vi "labVIEW_combinatie.vi"() -> ()   [LabVIEW 2019]
panel:
  in  "linksachter":bool
  in  "rechtsachter":bool
  in  "rechtsvooruit":bool
  in  "linksvooruit":bool
  in  "rechts":bool
  in  "links":bool
  out "port":u16
  in  "stop 2":bool
  out "data out":string
  in  "achteruit":bool
  in  "vooruit":bool
  in  "stop":bool
  # "sender"
  # "receiver"
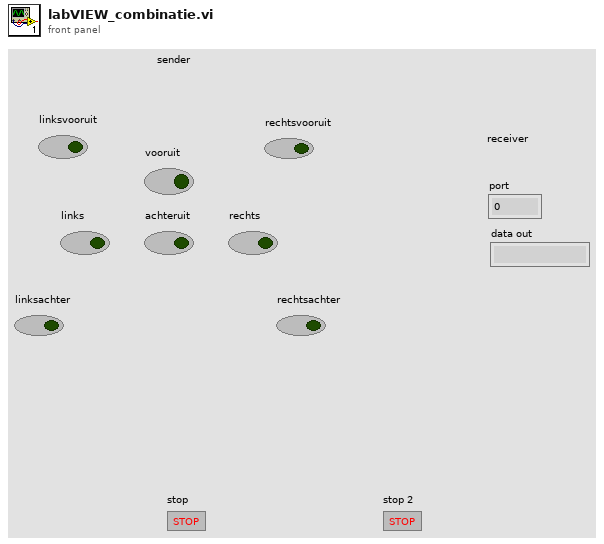
[diagram p1: front panel]
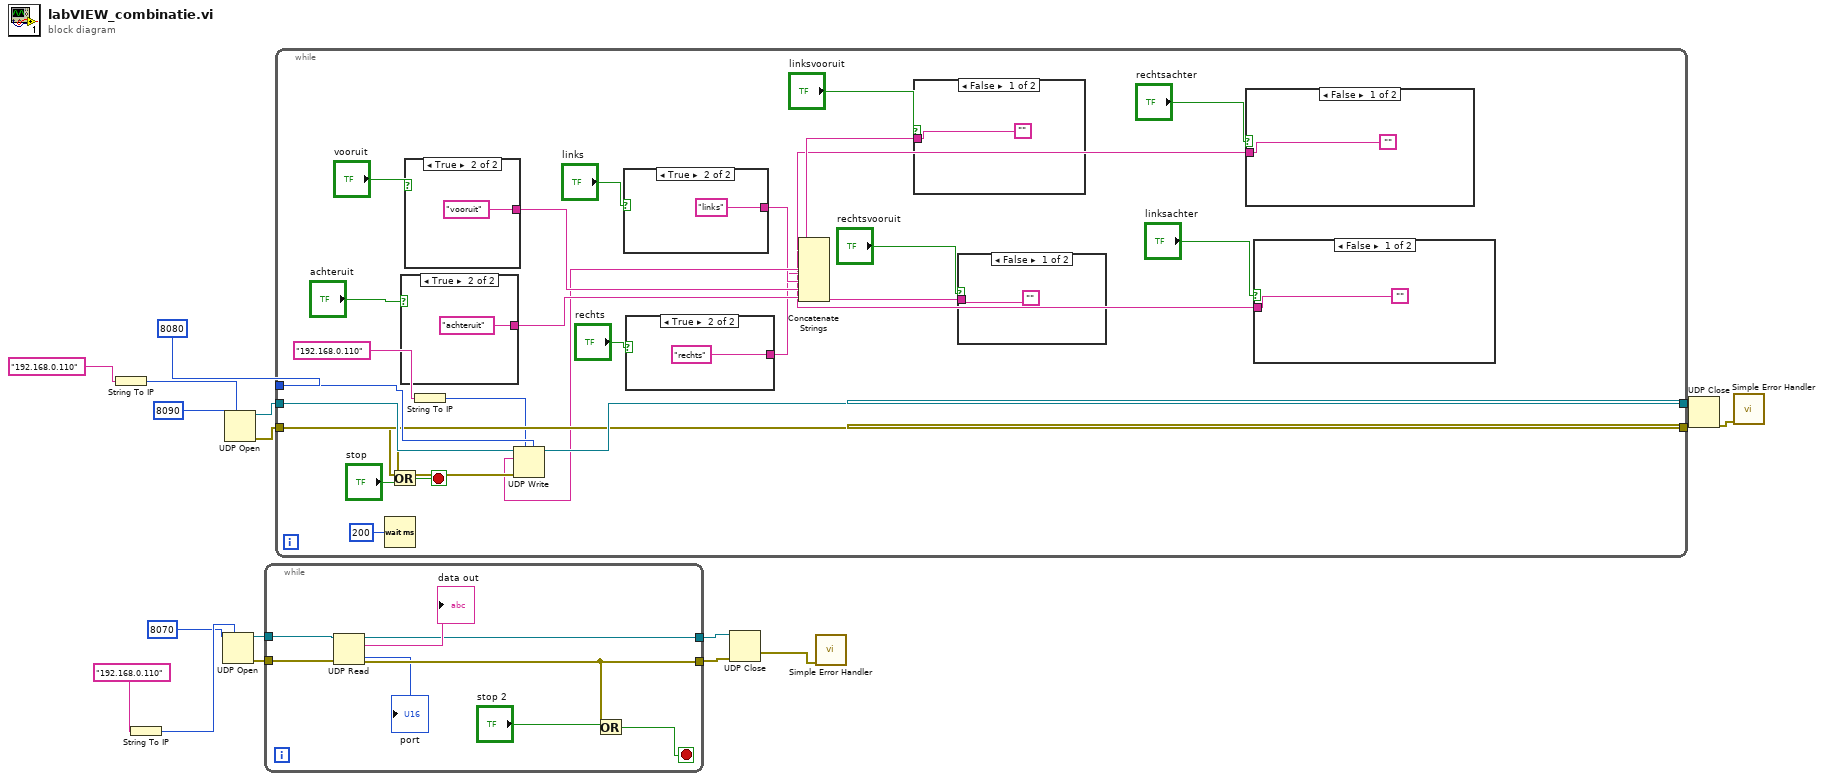
[diagram p0: block diagram]
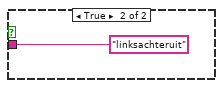
[diagram p2: hidden frame]
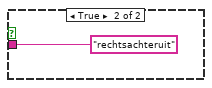
[diagram p3: hidden frame]
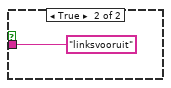
[diagram p4: hidden frame]
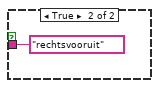
[diagram p5: hidden frame]
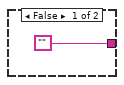
[diagram p6: hidden frame]
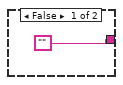
[diagram p7: hidden frame]
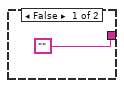
[diagram p8: hidden frame]
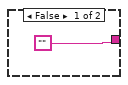
[diagram p9: hidden frame]
diagram:
  n1 = String To IP(1:"192.168.0.110") -> (0:w1:u32)
  n2 = String To IP(1:"192.168.0.110") -> (0:w7:u32)
  n3 = UDP Open(7:w7, 11:u16 8070 ("port")) -> (port=w5:refnum<k16>, 0:w4:errorcluster)  [unwired: 3 in, 1 out]
  n4 = UDP Open(7:w1, 11:8090) -> (port=w16:refnum<k16>, 0:w15:errorcluster)  [unwired: 3 in, 1 out]
  n5 = while {
    tunnel: [w22] -> w10
    tunnel: [w21] -> w9
    tunnel: w5 -> [w20]
    tunnel: w4 -> [w19]
    stop <- w23 stop-if-true
    n6 = UDP Read(connection ID=w20, 8:w19) -> (data out=→"data out":string, error out=w22:errorcluster, 3:w21:refnum<k16>, 4:→"port":u16)  [unwired: 2 in, 1 out]
    n7 = Or(x=w22, y="stop 2") -> (x .or. y?=w23:bool)
  }
  n8 = while {
    tunnel: w16 -> [w52]
    tunnel: w15 -> [w51]
    tunnel: 8080 -> [w47]
    tunnel: [w46] -> w13
    tunnel: [w45] -> w12
    stop <- w49 stop-if-true
    n9 = Wait (ms)(milliseconds to wait=200) -> ()  [unwired: 1 out]
    n10 = case shown="True" "achteruit" {
      tunnel: ["" "achteruit"] -> w41
      frame False {
      }
      frame True {
      }
    }
    n11 = case shown="True" "vooruit" {
      tunnel: ["" "vooruit"] -> w42
      frame False {
      }
      frame True {
      }
    }
    n12 = String To IP(1:"192.168.0.110") -> (0:w38:u32)
    n13 = case shown="True" "links" {
      tunnel: ["" "links"] -> w37
      frame False {
      }
      frame True {
      }
    }
    n14 = case shown="True" "rechts" {
      tunnel: ["" "rechts"] -> w35
      frame False {
      }
      frame True {
      }
    }
    n15 = case shown="False" "linksvooruit" {
      tunnel: ["" "linksvooruit"] -> w31
      frame False {
      }
      frame True {
      }
    }
    n16 = case shown="False" "rechtsvooruit" {
      tunnel: ["" "rechtsvooruit"] -> w32
      frame False {
      }
      frame True {
      }
    }
    n17 = case shown="False" "rechtsachter" {
      tunnel: ["" "rechtsachteruit"] -> w29
      frame False {
      }
      frame True {
      }
    }
    n18 = case shown="False" "linksachter" {
      tunnel: ["" "linksachteruit"] -> w28
      frame False {
      }
      frame True {
      }
    }
    n19 = Concatenate Strings(w28, w29, w31, w32, w35, w37, w42, w41) -> (w40:string)
    n20 = UDP Write(address=w38, port or service name=w47, connection ID=w52, data in=w40, 8:w51) -> (error out=w45:errorcluster, 3:w46:refnum<k16>)  [unwired: 1 in]
    n21 = Or(x=w45, y="stop") -> (x .or. y?=w49:bool)
  }
  n22 = UDP Close(connection ID=w9, 8:w10) -> (error out=w3:errorcluster)  [unwired: 1 out]
  n23 = call <vilib>:"Simple Error Handler.vi"("error in (no error)"=w3) -> ()  [unwired: 4 in, 5 out]
  n24 = UDP Close(connection ID=w13, 8:w12) -> (error out=w11:errorcluster)  [unwired: 1 out]
  n25 = call <vilib>:"Simple Error Handler.vi"("error in (no error)"=w11) -> ()  [unwired: 4 in, 5 out]
